vi "Add date info.vi"(8 "error in":errorcluster, 11 "Cluster in":T1={"Running VI"=refnum, "Test VI"=refnum, "Q Ref"=refnum, "UE"=refnum, "Data"=variant, "Timeout"=-1, "ListBox[]"=[], "Source Path"=path "", "Delta Time"=0.0, "ExifInfo[]"=[], "ListIndex"=0, "counter"=0, "Format"=enum."Files Only", "total"=0, "Operation"=enum."Read Info", "Status"=""} {"ExifInfo[]"."New DateTime" format="%<%.3X>T"; "ExifInfo[]"."DateTimeOrginal" format="%<%.3X>T"}) -> (0 "error out":errorcluster, 3 "Cluster out":T1={"Running VI"=refnum, "Test VI"=refnum, "Q Ref"=refnum, "UE"=refnum, "Data"=variant, "Timeout"=-1, "ListBox[]"=[], "Source Path"=path "", "Delta Time"=0.0, "ExifInfo[]"=[], "ListIndex"=0, "counter"=0, "Format"=enum."Files Only", "total"=0, "Operation"=enum."Read Info", "Status"=""} {"ExifInfo[]"."New DateTime" format="%<%.3X>T"; "ExifInfo[]"."DateTimeOrginal" format="%<%.3X>T"})   [LabVIEW 2023, in "EXIF Modifier.lvlib"]
uses:
  EXIF Modifier.lvlib
  Controls/exif_consumer cluster.ctl
  Controls/exif_info cluster.ctl
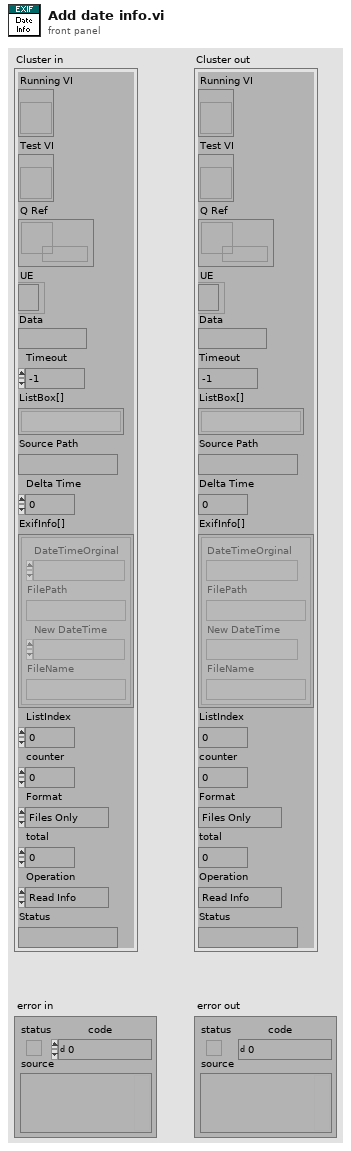
[diagram p1: front panel]
types:
  T1 = typedef "EXIF Modifier.lvlib/exif_consumer cluster.ctl" = cluster{"Running VI":refnum<vi>, "Test VI":refnum<vi>, "Q Ref":refnum<queue>, "UE":refnum<event-registration>, "Data":variant, "Timeout":i32, "ListBox[]":string[][], "Source Path":path, "Delta Time":dbl, "ExifInfo[]":T2[], "ListIndex":i32, "counter":i32, "Format":enum16{"Files Only", "Files Date", "All"}, "total":i32, "Operation":enum16{"Read Info", "Write Info"}, "Status":string}
  T2 = typedef "EXIF Modifier.lvlib/exif_info cluster.ctl" = cluster{"DateTimeOrginal":timestamp, "FilePath":path, "New DateTime":timestamp, "FileName":string}
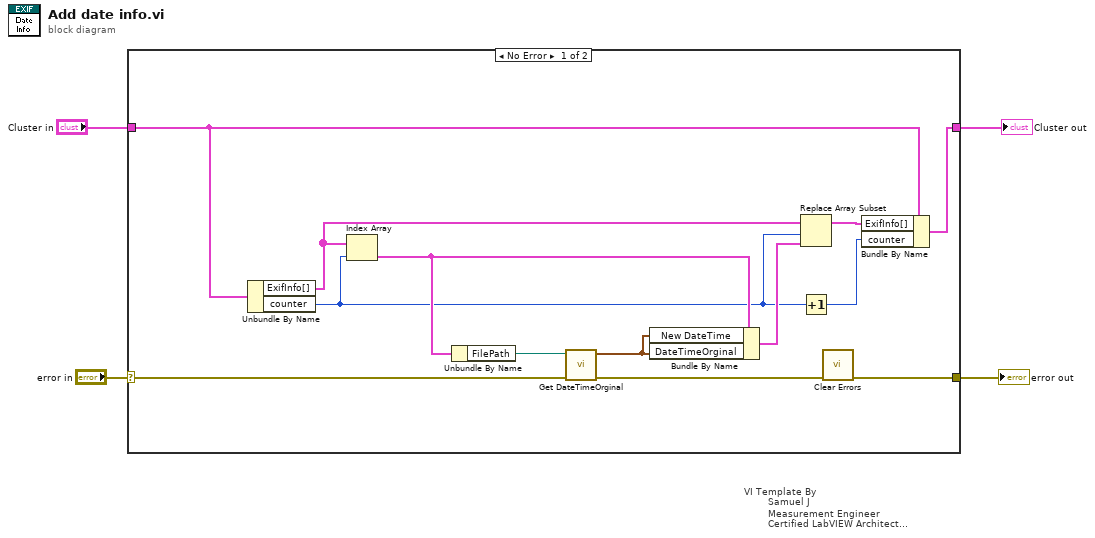
[diagram p0: block diagram]
diagram:
  n1 = case "VI Template By\n        Samuel J\n        Measurement Engineer\n        Certified LabVIEW Architect\n        Vestas Technology R&D Chennai" shown="No Error" "error in" {
    selector: "error in" -> [w15 w19]
    tunnel: [w6 w19] -> w3
    tunnel: [w16 w18] -> w1
    tunnel: "Cluster in" -> [w17 w18]
    frame No Error {
      n2 = Unbundle By Name(w17) -> ("ExifInfo[]"=w10:T2[], "counter"=w5:i32)
      n3 = Index Array(array=w10, index=w5) -> (element=w11:T2)
      n4 = Unbundle By Name(w11) -> ("FilePath"=w13:path)
      n5 = call "Get DateTimeOrginal.vi"("error in"=w15, "Path"=w13) -> ("error out"=w14:errorcluster, "output 1"=w12:timestamp)  [unwired: 7 in, 1 out]
      n6 = Bundle By Name(cluster=w11, "New DateTime"=w12, "DateTimeOrginal"=w12) -> (w9:T2)
      n7 = Replace Array Subset(array=w10, new element=w9, index=w5) -> (w8:T2[])
      n8 = Increment(x=w5) -> (x+1=w7:i32)
      n9 = call <vilib>:"Clear Errors.vi"("error in (no error)"=w14) -> ("error out"=w6:errorcluster)  [unwired: 5 in, 1 out]
      n10 = Bundle By Name(cluster=w17, "ExifInfo[]"=w8, "counter"=w7) -> (w16:T1)
    }
    frame Error {
    }
  }
  "error out" <- w3
  "Cluster out" <- w1
